vi "Main.vi"(8 "error in (no error)":errorcluster) -> (0 "error out":errorcluster)   [LabVIEW 2025]
uses:
  SubVIs/Controls/State_Machine_Ctrl.ctl
  SubVIs/Controls/TypeDef_FGV.ctl
  SubVIs/FGV/FGV_DO_Table.vi
  <vilib>/DAQmx/write.llb/DAQmx Write (Digital 1D U32 1Chan NSamp).vi
  <vilib>/DAQmx/write.llb/DAQmx Write (Analog 1D Wfm NChan NSamp).vi
panel:
  out "DO WF":waveform(i16)(graph)
  in  "sample mode":i32(ring)=10123 items=["Échantillons finis"=10178, "Échantillons continus"=10123, "Point par point avec cadencement matériel"=12522]
  in  "A02_voltage":dbl(slide)=-6.615384615384615 min=-10.0 max=10.0 step=0.1 scale=-10.0..10.0
  in  "A01_voltage":dbl(slide)=4.76923076923077 min=-10.0 max=10.0 step=0.1 scale=-10.0..10.0
  out "AO WF":waveform(dbl)[](graph)=[{"t0"=timestamp(0 s since 1904-01-01), "dt"=inf, "Y"=[]}, {"t0"=timestamp(0 s since 1904-01-01), "dt"=inf, "Y"=[]}]
  out "Dimension":u32
  in  "Readout time (s)":dbl=0.5
  in  "Exposure time (s)":dbl=0.1
  in  "Start":bool
  in  "Stop":bool
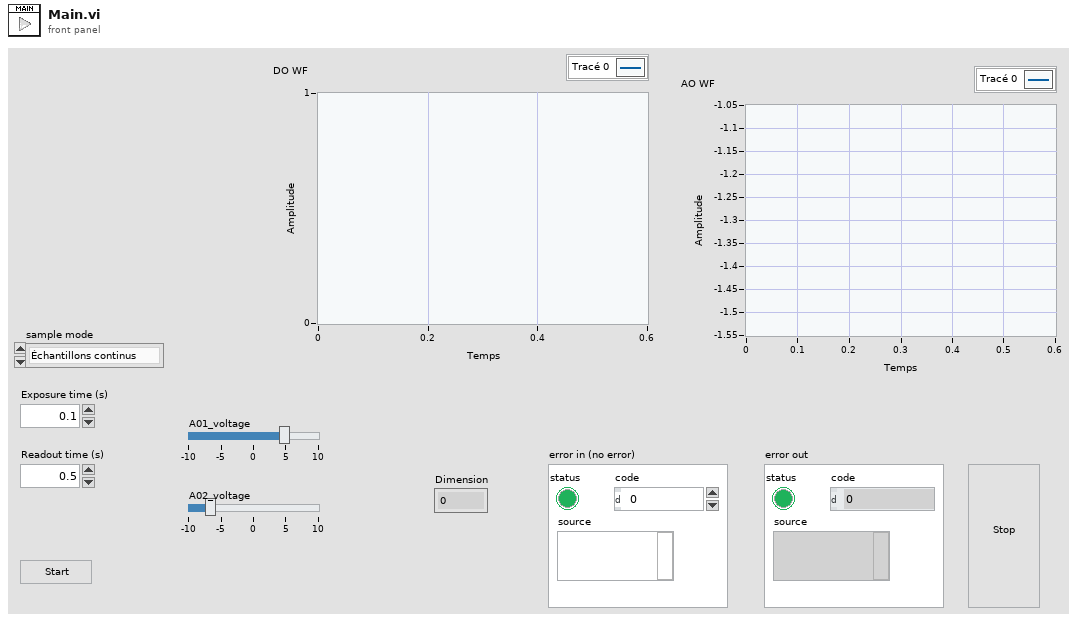
[diagram p1: front panel]
types:
  T1 = typedef "State_Machine_Ctrl.ctl" = enum16{"Initialize", "Wait for Event", "Setup_DAQ", "Create WF", "Generate WF", "Stop"}
  T2 = typedef "TypeDef_FGV.ctl" = enum16{"Initialize", "Write", "Read"}
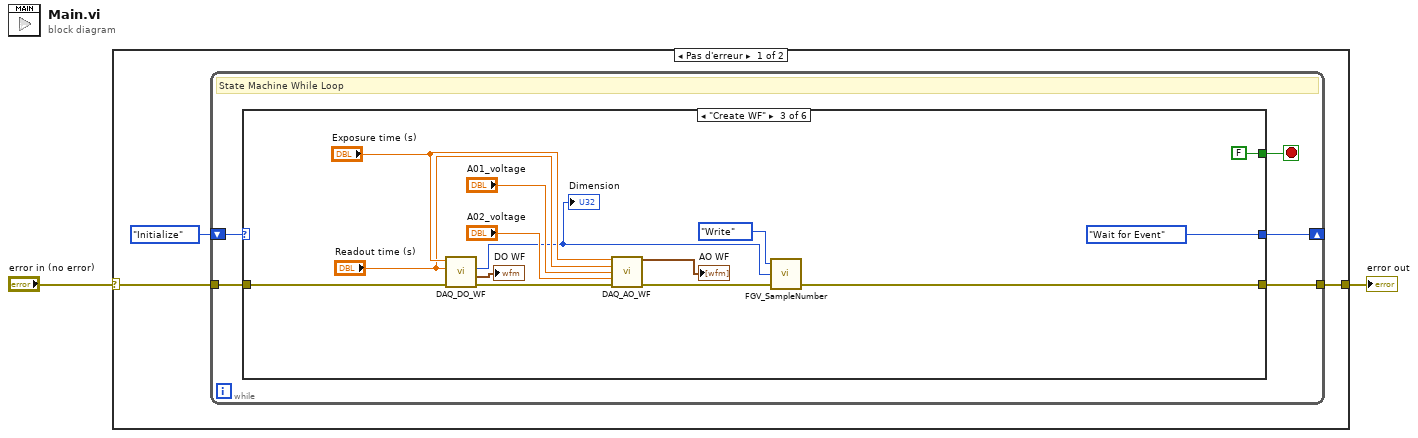
[diagram p0: block diagram]
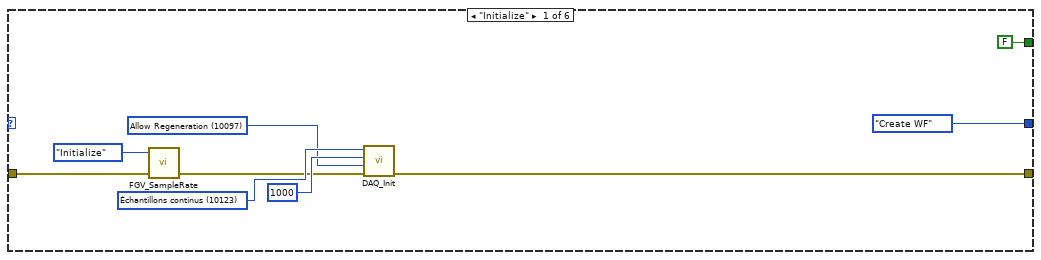
[diagram p2: hidden frame]
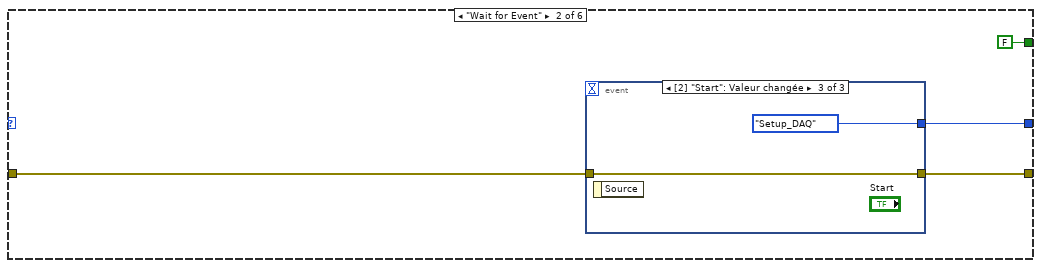
[diagram p3: hidden frame]
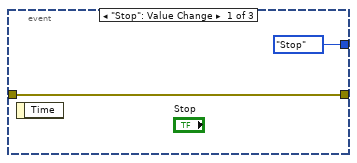
[diagram p4: hidden frame]
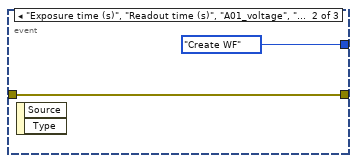
[diagram p5: hidden frame]
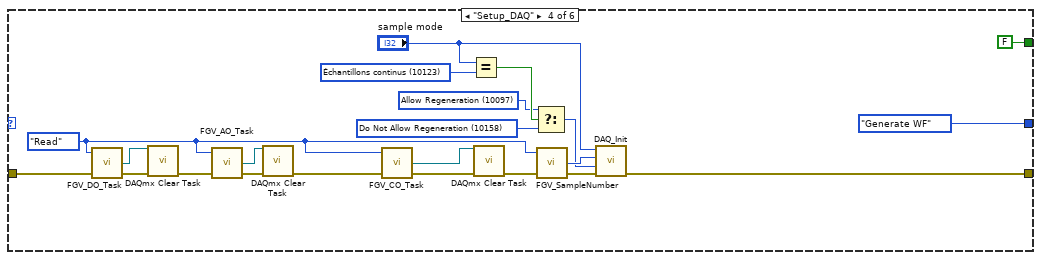
[diagram p6: hidden frame]
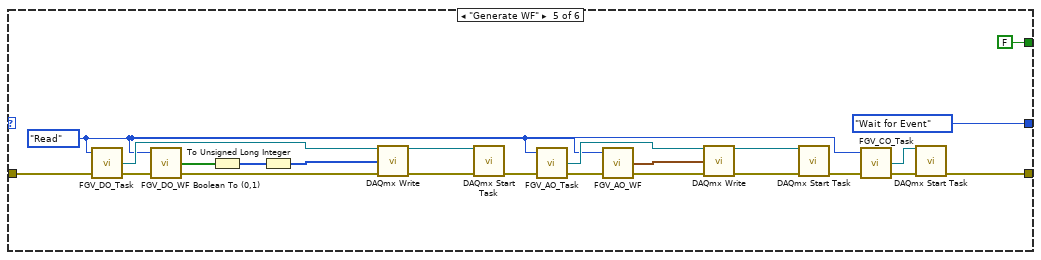
[diagram p7: hidden frame]
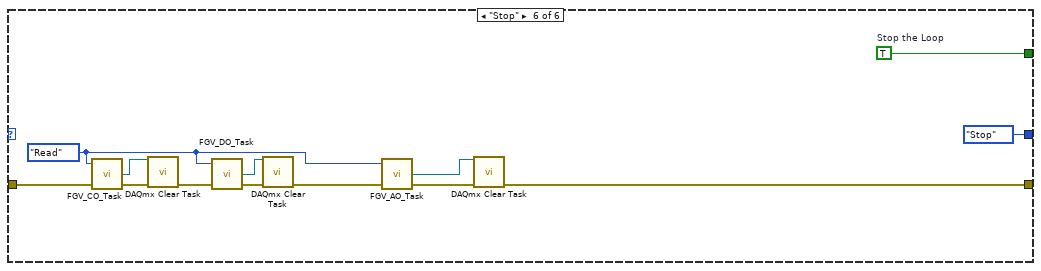
[diagram p8: hidden frame]
diagram:
  n1 = case shown="Pas d'erreur" "error in (no error)" {
    selector: "error in (no error)" -> [w4 w102]
    tunnel: [w3 w102] -> w2
    frame No Error {
      n2 = while {
        shift-right: [w9] -> _
        shift-left: State_Machine_Ctrl."Initialize" ("Initial State") -> [w10]
        tunnel: w4 -> [w7]
        tunnel: [w6] -> w3
        stop <- w8 stop-if-true
        # "State Machine While Loop"
        n3 = case "State Machine Case Structure" shown="\"Create WF\"" w10 {
          tunnel: [State_Machine_Ctrl."Create WF" ("Initial State") w23 State_Machine_Ctrl."Wait for Event" ("Initial State") State_Machine_Ctrl."Generate WF" ("Initial State") State_Machine_Ctrl."Wait for Event" ("Initial State") State_Machine_Ctrl."Stop" ("Initial State")] -> w9
          tunnel: [FALSE ("Stop the Loop") FALSE ("Stop the Loop") FALSE ("Stop the Loop") FALSE ("Stop the Loop") FALSE ("Stop the Loop") w101] -> w8
          tunnel: w7 -> [w16 w21 w41 w63 w85 w98]
          tunnel: [w12 w20 w32 w50 w69 w94] -> w6
          frame "Initialize" {
            w11 = 10097 items=["Allow Regeneration"=10097, "Do Not Allow Regeneration"=10158] ("RegenMode")
            w15 = 10123 items=["Échantillons finis"=10178, "Échantillons continus"=10123, "Point par point avec cadencement matériel"=12522] ("sample mode")
            # "Initialize - In this example, the only initialization required is to specify that the next state for the state machine is \"Wait for Event\"."
            n4 = call "FGV_SampleRate.vi"("error in"=w16, "Action"=TypeDef_FGV."Initialize") -> ("error out"=w13:errorcluster)  [unwired: 2 in, 1 out]
            n5 = call "DAQ_Init.vi"("error in"=w13, "RegenMode"=w11, "samples per channel"=1000, "sample mode"=w15) -> ("error out"=w12:errorcluster)  [unwired: 7 in]
          }
          frame "Wait for Event" {
            # "Wait for Event - An Event Structure is used to monitor the user interface for events. In each frame of the Event Structure, the next state of the state machine is specified based on which button was pressed."
            n6 = event shown="[2] \"Start\": Valeur changée" {
              selector: _ -> [_ _ _]
              dyn-events: _ -> [_ _ _]
              timeout: _ -> [_ _ _]
              tunnel: [State_Machine_Ctrl."Stop" ("Initial State") State_Machine_Ctrl."Create WF" ("Initial State") State_Machine_Ctrl."Setup_DAQ" ("Initial State")] -> w23
              tunnel: w21 -> [w24 w27 w28]
              tunnel: [w24 w27 w28] -> w20
              event "Stop": Value Change {
                n7 = event-data() -> ()  [unwired: 1 in, 1 out]
              }
              event "Exposure time (s)", "Readout time (s)", "A01_voltage", "A02_voltage": Value Change {
                n8 = event-data() -> ()  [unwired: 1 in, 2 out]
              }
              event "Start": Value Change {
                n9 = event-data() -> ()  [unwired: 1 in, 1 out]
              }
            }
          }
          frame "Create WF" {
            n10 = call "DAQ_DO_WF.vi"("error in"=w41, "Readout time (s)"="Readout time (s)", "Exposure time (s)"="Exposure time (s)") -> ("error out"=w31:errorcluster, "Graphe"=→"DO WF":waveform(i16), "Dimension"=w34:u32)  [unwired: 5 in, 1 out]
            "Dimension" <- w34
            n11 = call "DAQ_AO_WF.vi"("Exposure time (s)"="Exposure time (s)", "Readout time (s)"="Readout time (s)", "A01_voltage"="A01_voltage", "A02_voltage"="A02_voltage", "error in"=w31) -> ("AO WF"=→"AO WF":waveform(dbl)[], "error out"=w33:errorcluster)  [unwired: 8 in, 1 out]
            n12 = call "FGV_SampleNumber.vi"("error in"=w33, "Sample number"=w34, "Action"=TypeDef_FGV."Write") -> ("error out"=w32:errorcluster)  [unwired: 1 in, 1 out]
          }
          frame "Setup_DAQ" {
            w45 = 10158 items=["Allow Regeneration"=10097, "Do Not Allow Regeneration"=10158] ("RegenMode")
            w46 = 10097 items=["Allow Regeneration"=10097, "Do Not Allow Regeneration"=10158] ("RegenMode")
            w49 = 10123 items=["Échantillons finis"=10178, "Échantillons continus"=10123, "Point par point avec cadencement matériel"=12522] ("sample mode 2")
            w53 = TypeDef_FGV."Read" ("Action")
            n13 = call "FGV_DO_Task.vi"("error in"=w63, "Action"=w53) -> ("error out"=w62:errorcluster, "CO task"=w61:refnum<k21>)  [unwired: 2 in]
            n14 = call <vilib>:"DAQmx Clear Task.vi"("task in"=w61, "error in"=w62) -> ("error out"=w60:errorcluster)  [unwired: 13 in]
            n15 = call "FGV_AO_Task.vi"("error in"=w60, "Action"=w53) -> ("error out"=w59:errorcluster, "CO task"=w58:refnum<k21>)  [unwired: 2 in]
            n16 = call <vilib>:"DAQmx Clear Task.vi"("task in"=w58, "error in"=w59) -> ("error out"=w57:errorcluster)  [unwired: 13 in]
            n17 = call "FGV_CO_Task.vi"("error in"=w57, "Action"=w53) -> ("error out"=w56:errorcluster, "CO task"=w55:refnum<k21>)  [unwired: 2 in]
            n18 = Equal?(x="sample mode", y=w49) -> (x = y?=w48:bool)
            n19 = call <vilib>:"DAQmx Clear Task.vi"("task in"=w55, "error in"=w56) -> ("error out"=w54:errorcluster)  [unwired: 13 in]
            n20 = Select(t=w46, s=w48, f=w45) -> (s? t:f=w44:i32)
            n21 = call "FGV_SampleNumber.vi"("error in"=w54, "Action"=w53) -> ("error out"=w51:errorcluster, "Sample number"=w52:u32)  [unwired: 2 in]
            n22 = call "DAQ_Init.vi"("error in"=w51, "RegenMode"=w44, "samples per channel"=w52, "sample mode"="sample mode") -> ("error out"=w50:errorcluster)  [unwired: 7 in]
          }
          frame "Generate WF" {
            w71 = TypeDef_FGV."Read" ("Action")
            n23 = call "FGV_DO_Task.vi"("error in"=w85, "Action"=w71) -> ("error out"=w82:errorcluster, "CO task"=w84:refnum<k21>)  [unwired: 2 in]
            n24 = call "FGV_DO_WF.vi"("error in"=w82, "Action"=w71) -> ("error out"=w83:errorcluster, "DO table"=w68:bool[])  [unwired: 2 in]
            n25 = Boolean To (0,1)(Boolean=w68) -> (0, 1=w66:i16[])
            n26 = To Unsigned Long Integer(number=w66) -> (unsigned 32bit integer=w67:u32[])
            n27 = call-poly <vilib>:"DAQmx Write.vi"("task/channels in"=w84, "data"=w67, "error in"=w83) -> ("task out"=w80:refnum<k21>, "error out"=w79:errorcluster)  [unwired: 10 in, 1 out]
            n28 = call <vilib>:"DAQmx Start Task.vi"("task/channels in"=w80, "error in"=w79) -> ("error out"=w78:errorcluster)  [unwired: 12 in, 1 out]
            n29 = call "FGV_AO_Task.vi"("error in"=w78, "Action"=w71) -> ("error out"=w75:errorcluster, "CO task"=w81:refnum<k21>)  [unwired: 2 in]
            n30 = call "FGV_AO_WF.vi"("error in 2"=w75, "Action 2"=w71) -> ("error out 2"=w74:errorcluster, "AO WF 2"=w73:waveform(dbl)[])  [unwired: 2 in]
            n31 = call-poly <vilib>:"DAQmx Write.vi"("task/channels in"=w81, "data"=w73, "error in"=w74) -> ("task out"=w76:refnum<k21>, "error out"=w77:errorcluster)  [unwired: 10 in, 1 out]
            n32 = call <vilib>:"DAQmx Start Task.vi"("task/channels in"=w76, "error in"=w77) -> ("error out"=w70:errorcluster)  [unwired: 12 in, 1 out]
            n33 = call "FGV_CO_Task.vi"("error in"=w70, "Action"=w71) -> ("error out"=w72:errorcluster, "CO task"=w86:refnum<k21>)  [unwired: 2 in]
            n34 = call <vilib>:"DAQmx Start Task.vi"("task/channels in"=w86, "error in"=w72) -> ("error out"=w69:errorcluster)  [unwired: 12 in, 1 out]
          }
          frame "Stop" {
            w99 = TypeDef_FGV."Read" ("Action")
            w101 = TRUE  # Stop the Loop
            # "Stop - Stop the VI. This is the only state that specifies a TRUE value for the loop conditional terminal."
            n35 = call "FGV_CO_Task.vi"("error in"=w98, "Action"=w99) -> ("error out"=w96:errorcluster, "CO task"=w97:refnum<k21>)  [unwired: 2 in]
            n36 = call <vilib>:"DAQmx Clear Task.vi"("task in"=w97, "error in"=w96) -> ("error out"=w95:errorcluster)  [unwired: 13 in]
            n37 = call "FGV_DO_Task.vi"("error in"=w95, "Action"=w99) -> ("error out"=w91:errorcluster, "CO task"=w90:refnum<k21>)  [unwired: 2 in]
            n38 = call <vilib>:"DAQmx Clear Task.vi"("task in"=w90, "error in"=w91) -> ("error out"=w92:errorcluster)  [unwired: 13 in]
            n39 = call "FGV_AO_Task.vi"("error in"=w92, "Action"=w99) -> ("error out"=w93:errorcluster, "CO task"=w89:refnum<k21>)  [unwired: 2 in]
            n40 = call <vilib>:"DAQmx Clear Task.vi"("task in"=w89, "error in"=w93) -> ("error out"=w94:errorcluster)  [unwired: 13 in]
          }
        }
      }
    }
    frame Error {
    }
  }
  "error out" <- w2
